vi "List COM port.vi"(8 "error in (no error)":errorcluster) -> (0 "error out":errorcluster, 3 "COM Ports":string[](array[string]))   [LabVIEW 2013, in "Thorlabs_FWxC.lvlib"]
doc: "Establishes communication with the instrument and optionally performs an instrument identification query and/or an instrument reset. It also places the instrument in a default state needed for other instrument driver operations. Therefore, call this VI before calling other instrument driver VIs for this instrument. Generally, you need to call the Initialize VI only once at the beginning of an application."
uses:
  <instrlib>/Thorlabs_FWxC/Thorlabs_FWxC.lvlib
  <instrlib>/Thorlabs_FWxC/Library/FilterWheel102_win32.dll
  <instrlib>/Thorlabs_FWxC/Library/FilterWheel102_win64.dll
panel:
  out "return type":i32
  # "(c) 2020 <Thorlabs>.  ALL RIGHTS RESERVED."
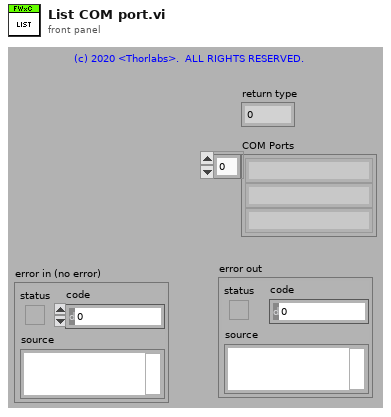
[diagram p1: front panel]
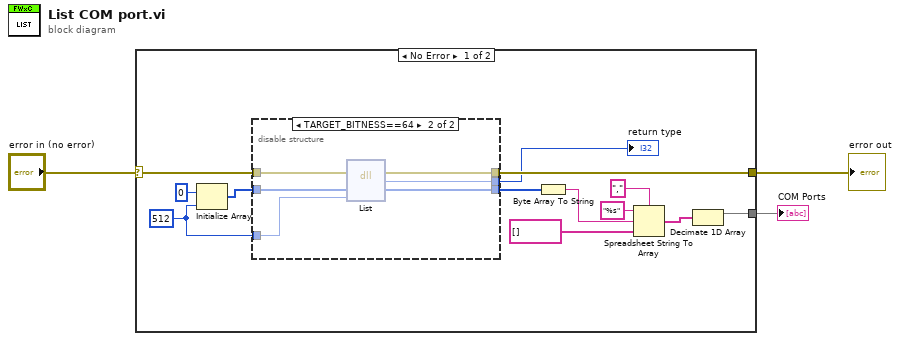
[diagram p0: block diagram]
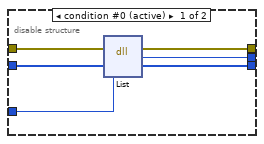
[diagram p2: hidden frame]
diagram:
  n1 = case shown="No Error" "error in (no error)" {
    selector: "error in (no error)" -> [w16 w29]
    tunnel: [w15 w29] -> w3
    tunnel: [w10 _] -> w1
    frame No Error {
      w4 = 512 ("dimension size")
      n2 = Initialize Array(u8 0 ("element"), w4) -> (w7:u8[])
      n3 = disable-structure shown="TARGET_BITNESS==64" {
        disable-tunnel: w16 -> [w22 w28]
        disable-tunnel: [w21 w27] -> w15
        disable-tunnel: [w20 w25] -> w9
        disable-tunnel: w7 -> [w19 w26]
        disable-tunnel: [w18 w24] -> w5
        disable-tunnel: w4 -> [w17 w23]
        frame condition #0 (active) {
          n4 = dll-call lib="C:/Program Files (x86)/National Instruments/LabVIEW 2013/instr.lib/Thorlabs_FWxC/Library/FilterWheel102_win32.dll" fn="List"(error in=w22, "ports"=w19, "length"=w17) -> (error out=w21:errorcluster, "return type"=w18:i32, "ports"=w20:u8[])  [unwired: 3 in, 1 out]
        }
        frame condition #1 {
          n5 = dll-call lib="C:/Program Files/National Instruments/LabVIEW 2013/instr.lib/Thorlabs_FWxC/Library/FilterWheel102_win64.dll" fn="List"(error in=w28, "ports"=w26, "length"=w23) -> (error out=w27:errorcluster, "return type"=w24:i32, "ports"=w25:u8[])  [unwired: 3 in, 1 out]
        }
      }
      "return type" <- w5
      n6 = Byte Array To String(unsigned byte array=w9) -> (string=w6:string)
      n7 = Spreadsheet String To Array(delimiter (Tab)=",", format string="%s", spreadsheet string=w6, array type (2D Dbl)=string[] []) -> (array=w11:string[])
      n8 = Decimate 1D Array(w11) -> (w10:string[])  [unwired: 1 out]
    }
    frame Error {
    }
  }
  "error out" <- w3
  "COM Ports" <- w1
